vi "Get (U32).vi"(11 "Value in":refnum<class "Value.lvclass">) -> (1 "Is Defined?":bool, 2 "Value":u32, 3 "Value out":refnum<class "Value.lvclass">)   [LabVIEW 2024, in "EDS.lvlib" / "Value.lvclass"]
uses:
  Value.lvclass
  Value.lvclass/Value.ctl
  EDS.lvlib
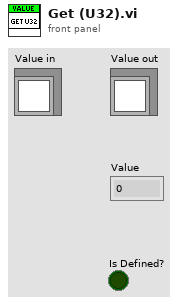
[diagram p1: front panel]
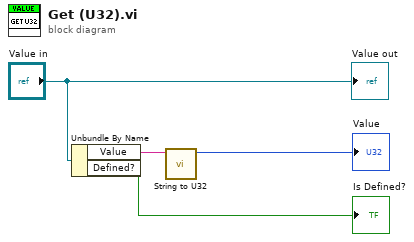
[diagram p0: block diagram]
diagram:
  n1 = Unbundle By Name("Value in") -> ("Value"=w3:string, "Defined?"=→"Is Defined?":bool)
  n2 = call "String to U32.vi"("String"=w3) -> ("U32"=→"Value":u32)  [unwired: 10 in]
  "Value out" <- "Value in"
